vi "4_Select Elements from Array_solution.vi"(8 "Max":dbl=5.0, 9 "Min":dbl=2.0, 11 "Input Array":dbl[][](array[numeric])=[[5.0, 3.0, 1.0], [10.0, 59.0, 12.0], [33.0, 2.0, 39.0], [91.0, 7.0, 10.0], [7.0, 8.0, 25.0]]) -> (2 "Result: Elements Out of Range":dbl[](array[numeric]))   [LabVIEW 2014]
panel:
  # "Numbers in the Input Array will be filetered according to\nthe range give by the Min and Max Control\nResult Number is out of range given by Min and Max\nResult Number<Min\nResult Number>Max\nSee the following example"
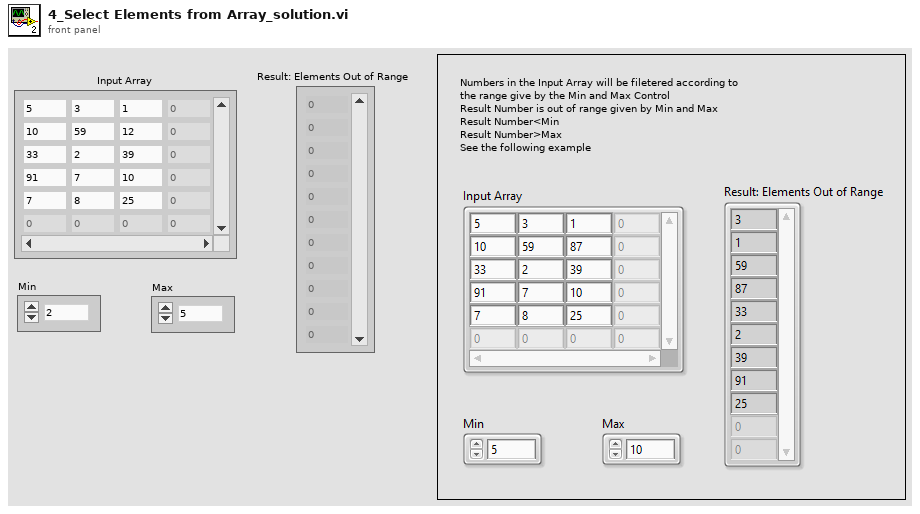
[diagram p1: front panel]
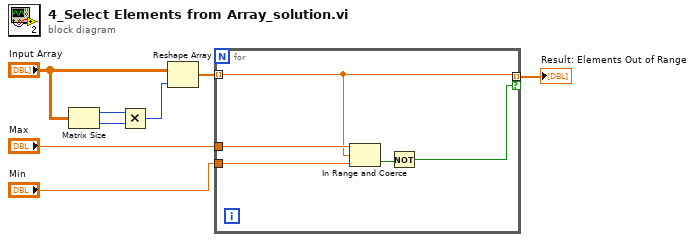
[diagram p0: block diagram]
diagram:
  n1 = Matrix Size(0:"Input Array") -> (1:w6:i32, 2:w7:i32)
  n2 = Multiply(x=w6, y=w7) -> (x*y=w5:i32)
  n3 = Reshape Array("Input Array", w5) -> (w4:dbl[])
  n4 = for {
    tunnel: [w11] -> w1 mode=indexing if=w9
    tunnel: w4 -> [w11] mode=indexing
    tunnel: "Max" -> [w13]
    tunnel: "Min" -> [w12]
    n5 = In Range and Coerce(upper limit=w13, x=w11, lower limit=w12) -> (In Range?=w10:bool)  [unwired: 1 out]
    n6 = Not(x=w10) -> (.not. x?=w9:bool)
  }
  "Result: Elements Out of Range" <- w1
